vi "AlGaInPAs_prep_run_cont_v06.vi"(2 "Debug Mode":bool, 3 "Elapsed Time(s)":dbl, 4 "State":enum16{"Edit", "Start", "Run", "End", "Idle"}(ring), 5 "Argument List In":string[](array[string])) -> (0 "Status Out":string, 1 "Argument List Out":string[](array[string]))   [LabVIEW 2011]
panel:
  out "first":bool=TRUE
  out "total time":dbl
  out "is OK?":bool
  out "AsH3?":bool
  out "PH3?":bool
  out "In?":bool
  out "Ga?":bool
  out "Al?":bool
  in  "Prep As":bool caption="Pre-run"
  in  "Prep P":bool caption="Pre-run"
  in  "Prep In":bool caption="Pre-run"
  in  "Prep Ga":bool caption="Pre-run"
  in  "prep_time":dbl caption="pre-run time (s)"
  in  "Prep Al":bool caption="Pre-run"
  in  "Run As":bool caption="Run"
  in  "AsH3 Flow":dbl caption="AsH3 Flow (0-10 sccm)" format="%.2f"
  in  "P Flow":dbl caption="P Flow (0-100 sccm)" format="%.2f"
  in  "Run P":bool caption="Run"
  in  "In Flow":dbl caption="In Flow (0-100 sscm)" format="%.2f"
  in  "Run In":bool caption="Run"
  in  "Run Ga":bool caption="Run"
  in  "Ga Flow":dbl caption="Ga Flow (0-10 sscm)" format="%.2f"
  in  "Run Al":bool caption="Run"
  in  "Al Flow":dbl caption="Al Flow (0-100 sscm)" format="%.2f"
  in  "Cancel":bool
  in  "OK":bool
  out "tTotal(s) 2":dbl
  # "Add pre-run time to run time in editor."
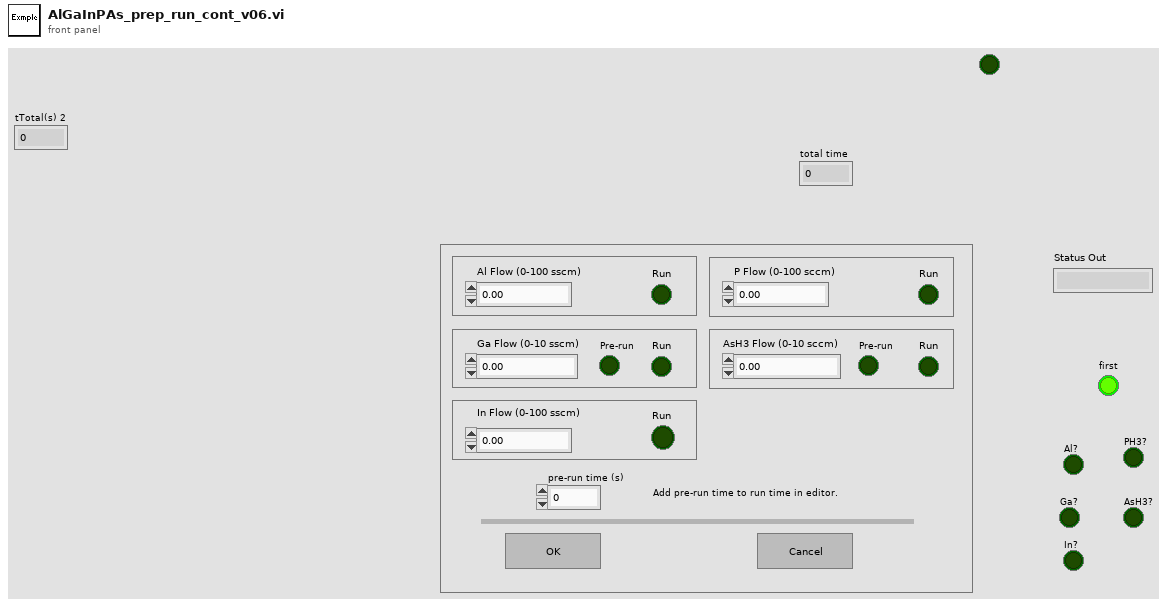
[diagram p1: front panel]
types:
  T1 = enum16{"Discrete", "Continuous", "Instantaneous"}
  T2 = enum32{"Invalid", "Default", "Floating", "Floating/Auto-Hide", "Modal"}
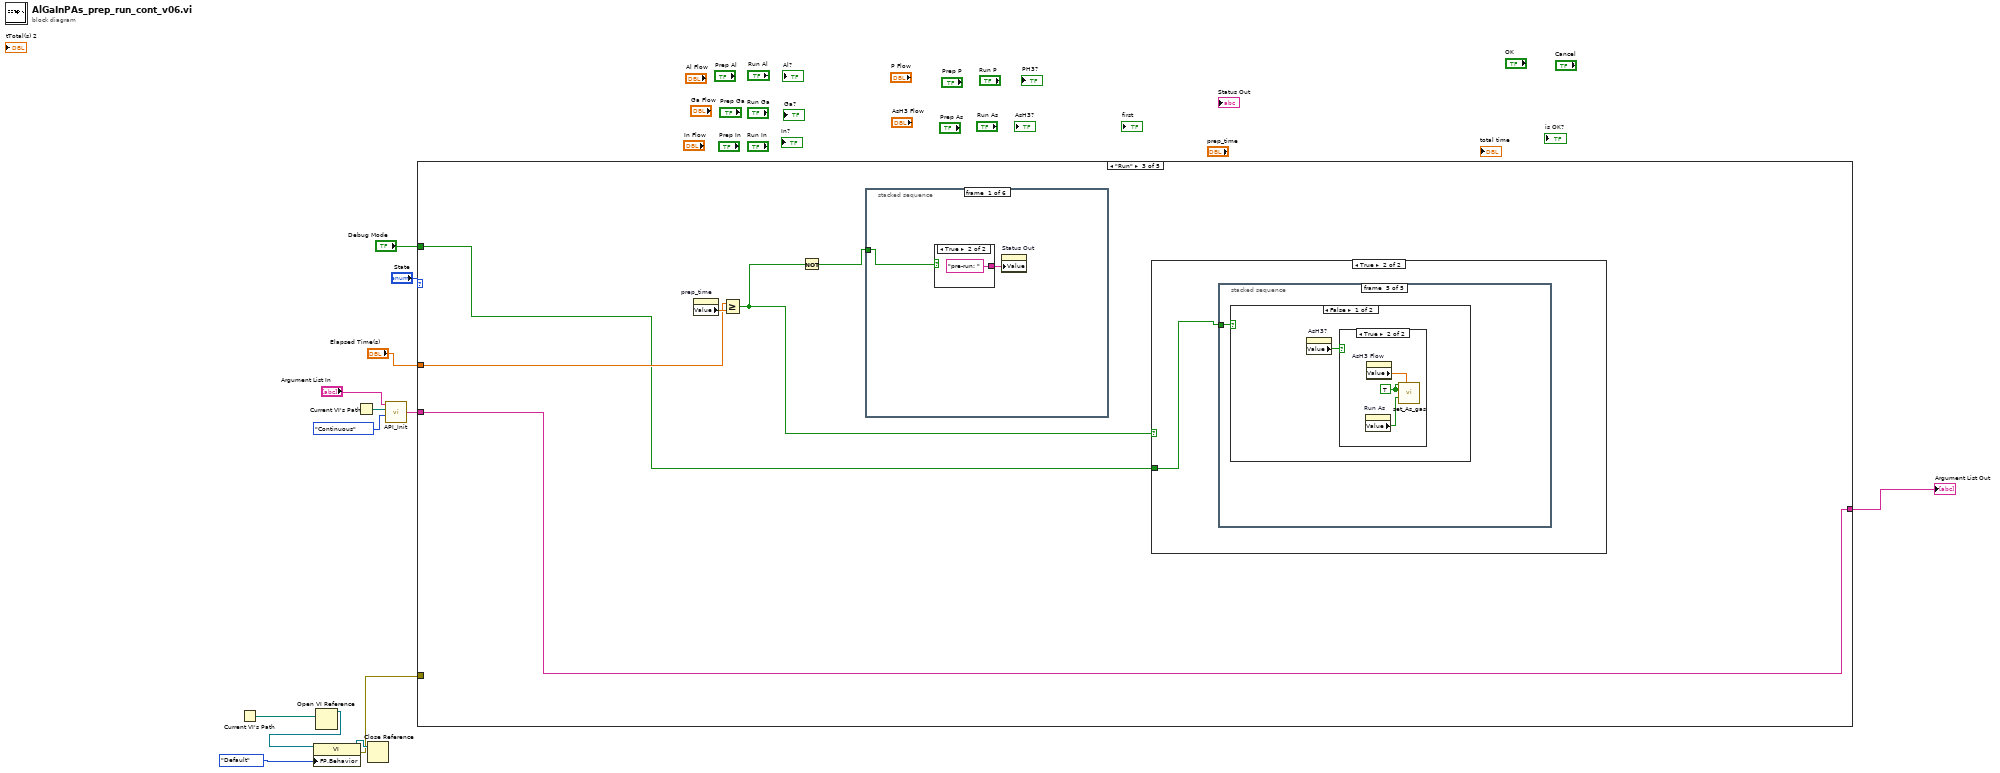
[diagram p0: block diagram]
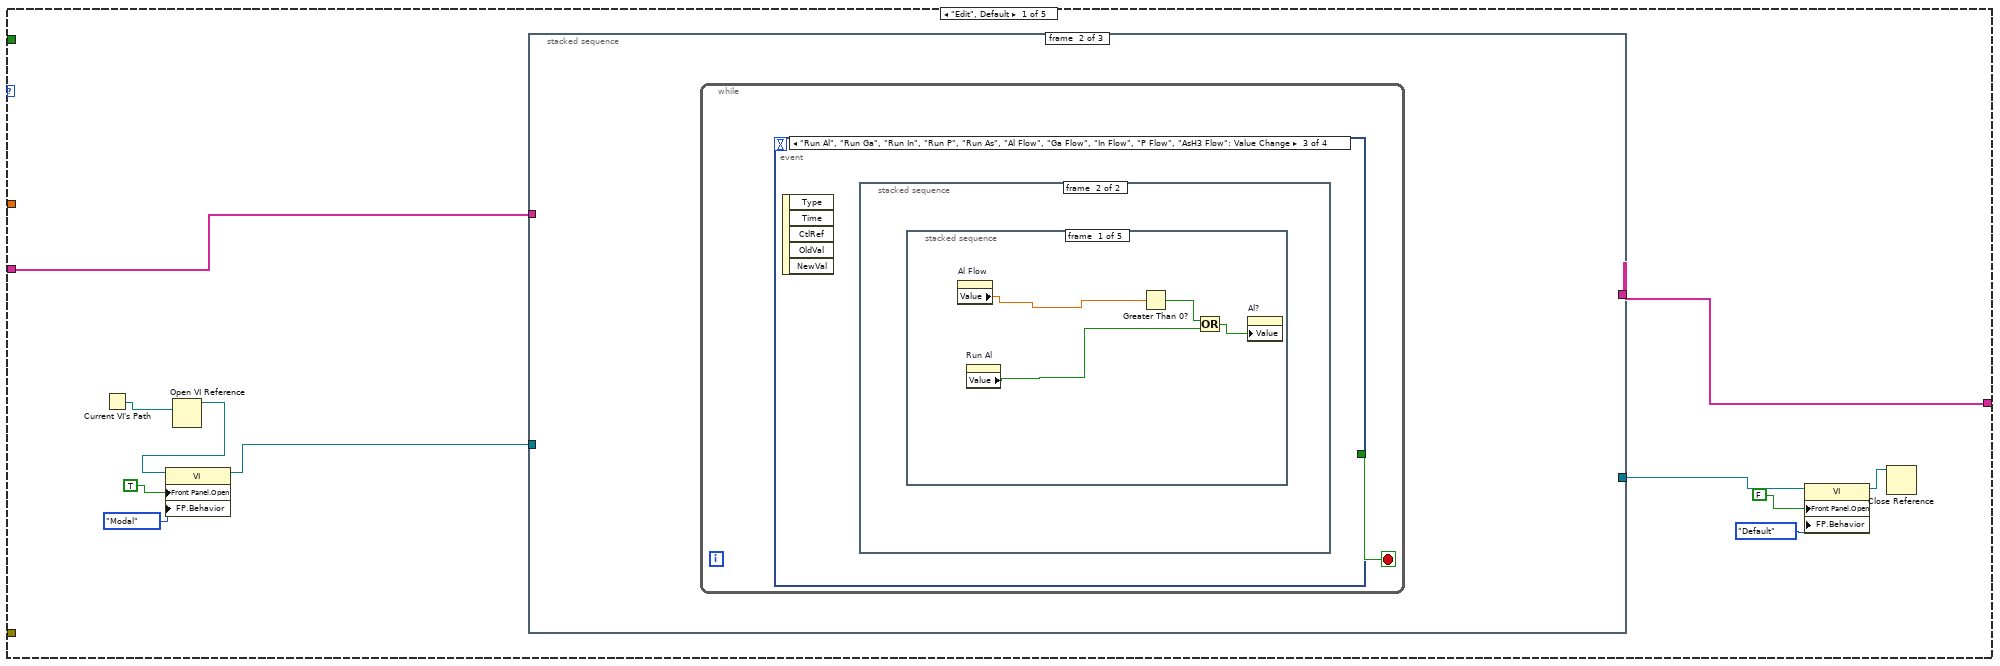
[diagram p2: hidden frame]
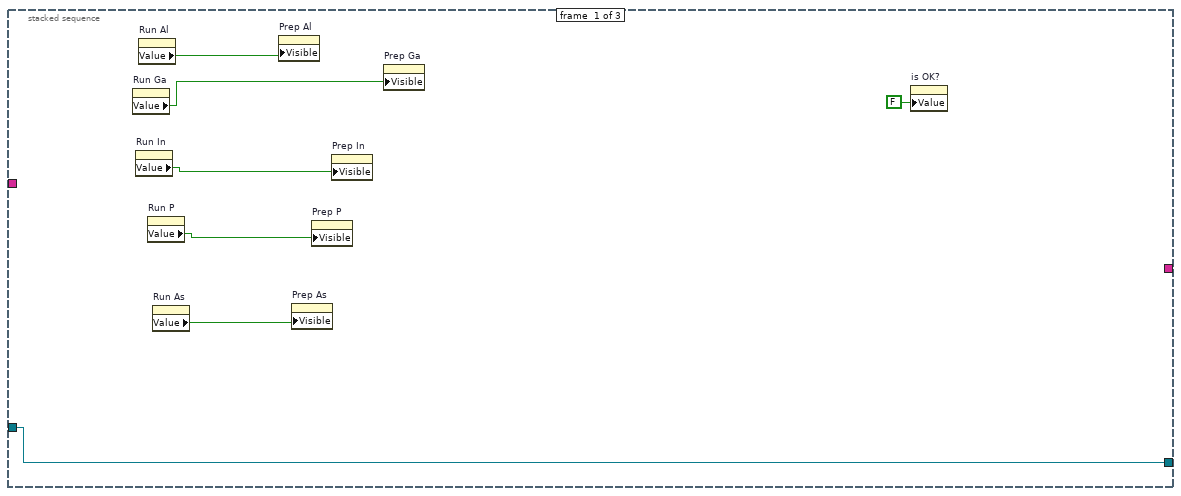
[diagram p3: hidden frame]
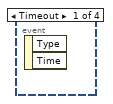
[diagram p4: hidden frame]
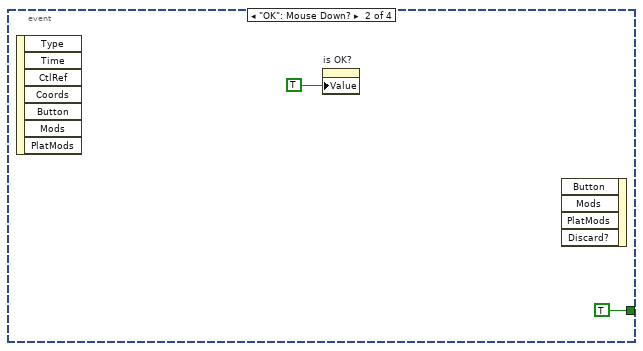
[diagram p5: hidden frame]
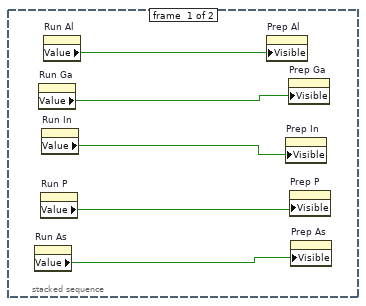
[diagram p6: hidden frame]
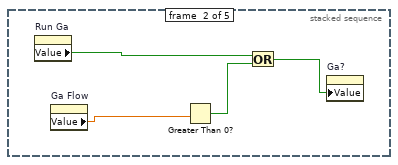
[diagram p7: hidden frame]
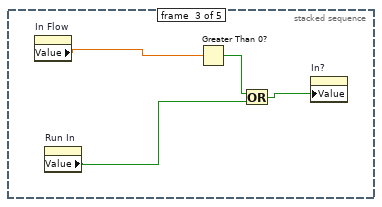
[diagram p8: hidden frame]
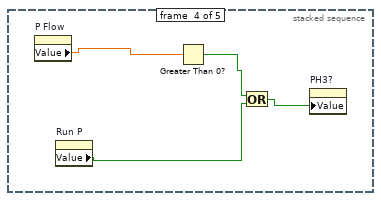
[diagram p9: hidden frame]
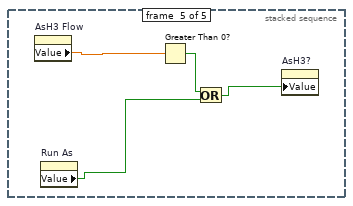
[diagram p10: hidden frame]
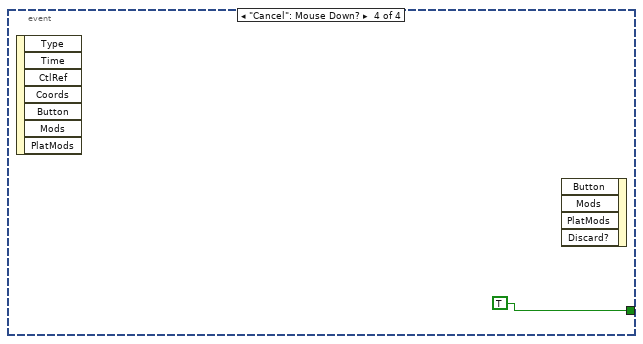
[diagram p11: hidden frame]
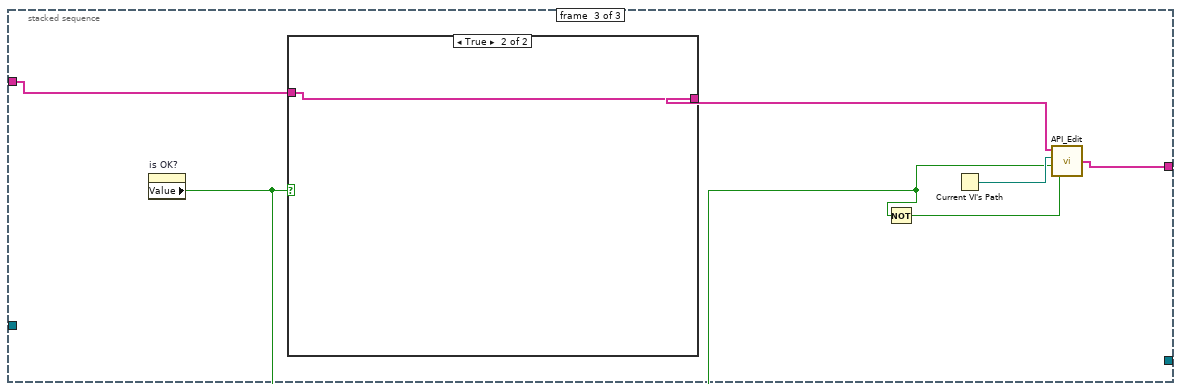
[diagram p12: hidden frame]
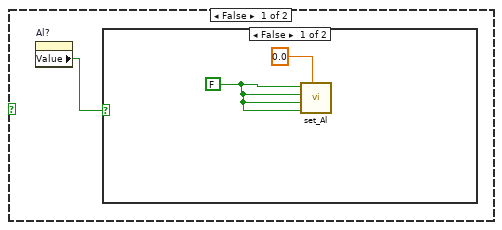
[diagram p15: hidden frame]
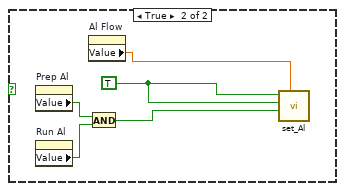
[diagram p16: hidden frame]
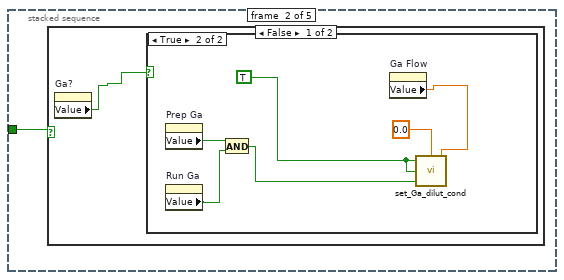
[diagram p17: hidden frame]
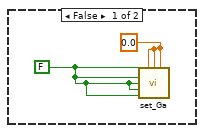
[diagram p18: hidden frame]
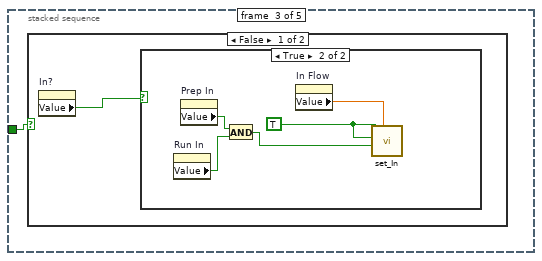
[diagram p20: hidden frame]
diagram:
  n1 = Current VI's Path() -> (path=w9:path)
  n2 = Open VI Reference(vi path=w9) -> (vi reference=w8:refnum<vi>)  [unwired: 1 in, 5 out]
  n3 = property class="VI"(reference=w8, "FP.Behavior"=T2."Default" ("Front Panel Window:Behavior")) -> (reference out=w6:refnum<vi>, error out=w5:errorcluster)  [unwired: 1 in]
  n4 = Current VI's Path() -> (path=w4:path)
  n5 = Close Reference(reference=w6) -> ()  [unwired: 1 in, 1 out]
  n6 = call "API_Init.vi"("API Mode"=T1."Continuous", "VI Path"=w4, "Argument List In"="Argument List In") -> ("Argument List Out"=w1:string[])  [unwired: 1 in]
  n7 = case shown="\"Run\"" "State" {
    tunnel: "Debug Mode" -> [_ w69 w120 _ _]
    tunnel: "Elapsed Time(s)" -> [_ _ w121 _ _]
    tunnel: w1 -> [w15 w70 w123 w210 w211]
    tunnel: [w14 w70 w123 w210 w211] -> w10
    tunnel: w5 -> [_ _ _ _ _]
    frame "Edit", Default {
      n8 = Current VI's Path() -> (path=w20:path)
      n9 = Open VI Reference(vi path=w20) -> (vi reference=w19:refnum<vi>)  [unwired: 1 in, 5 out]
      n10 = property class="VI"(reference=w19, "Front Panel.Open"=TRUE ("Front Panel Window:Open"), "FP.Behavior"=T2."Modal" ("Front Panel Window:Behavior")) -> (reference out=w18:refnum<vi>)  [unwired: 1 in, 1 out]
      n11 = stacked-sequence {
        tunnel: w15 -> [_ _ w64]
        tunnel: w18 -> [w31 _ _]
        tunnel: [w31 _ _] -> w22
        tunnel: [_ _ w62] -> w14
        frame #0 {
          n12 = property on="Run Ga" class="Bool (strict)"() -> ("Value"=w28:bool)  [unwired: 2 in, 2 out]
          n13 = property on="Run In" class="Bool (strict)"() -> ("Value"=w27:bool)  [unwired: 2 in, 2 out]
          n14 = property on="Run Al" class="Bool (strict)"() -> ("Value"=w29:bool)  [unwired: 2 in, 2 out]
          n15 = property on="Run P" class="Bool (strict)"() -> ("Value"=w26:bool)  [unwired: 2 in, 2 out]
          n16 = property on="Run As" class="Bool (strict)"() -> ("Value"=w25:bool)  [unwired: 2 in, 2 out]
          n17 = property on="Prep Al" class="Bool (strict)"("Visible"=w29) -> ()  [unwired: 2 in, 2 out]
          n18 = property on="Prep As" class="Bool (strict)"("Visible"=w25) -> ()  [unwired: 2 in, 2 out]
          n19 = property on="Prep P" class="Bool (strict)"("Visible"=w26) -> ()  [unwired: 2 in, 2 out]
          n20 = property on="Prep In" class="Bool (strict)"("Visible"=w27) -> ()  [unwired: 2 in, 2 out]
          n21 = property on="Prep Ga" class="Bool (strict)"("Visible"=w28) -> ()  [unwired: 2 in, 2 out]
          n22 = property on="is OK?" class="Bool (strict)"("Value"=FALSE ("is OK?")) -> ()  [unwired: 2 in, 2 out]
        }
        frame #1 {
          n23 = while {
            stop <- w32 stop-if-true
            n24 = event shown="[2] \"Run Al\", \"Run Ga\", \"Run In\", \"Run P\", \"Run As\", \"Al Flow\", \"Ga Flow\", \"In Flow\", \"P Flow\", \"AsH3 Flow\": Value Change" {
              selector: _ -> [_ _ _ _]
              dyn-events: _ -> [_ _ _ _]
              timeout: _ -> [_ _ _ _]
              tunnel: [_ TRUE _ TRUE] -> w32
              event Timeout {
                n25 = event-data() -> ()  [unwired: 1 in, 2 out]
              }
              event "OK": Mouse Down? {
                n26 = event-data() -> ()  [unwired: 1 in, 7 out]
                n27 = property on="is OK?" class="Bool (strict)"("Value"=TRUE ("is OK?")) -> ()  [unwired: 2 in, 2 out]
                n28 = event-data() -> ()  [unwired: 5 in, 1 out]
              }
              event "Run Al", "Run Ga", "Run In", "Run P", "Run As", "Al Flow", "Ga Flow", "In Flow", "P Flow", "AsH3 Flow": Value Change {
                n29 = event-data() -> ()  [unwired: 1 in, 5 out]
                n30 = stacked-sequence {
                  frame #0 {
                    n31 = property on="Run As" class="Bool (strict)"() -> ("Value"=w35:bool)  [unwired: 2 in, 2 out]
                    n32 = property on="Run Ga" class="Bool (strict)"() -> ("Value"=w38:bool)  [unwired: 2 in, 2 out]
                    n33 = property on="Run P" class="Bool (strict)"() -> ("Value"=w36:bool)  [unwired: 2 in, 2 out]
                    n34 = property on="Run In" class="Bool (strict)"() -> ("Value"=w37:bool)  [unwired: 2 in, 2 out]
                    n35 = property on="Run Al" class="Bool (strict)"() -> ("Value"=w39:bool)  [unwired: 2 in, 2 out]
                    n36 = property on="Prep Al" class="Bool (strict)"("Visible"=w39) -> ()  [unwired: 2 in, 2 out]
                    n37 = property on="Prep In" class="Bool (strict)"("Visible"=w37) -> ()  [unwired: 2 in, 2 out]
                    n38 = property on="Prep Ga" class="Bool (strict)"("Visible"=w38) -> ()  [unwired: 2 in, 2 out]
                    n39 = property on="Prep P" class="Bool (strict)"("Visible"=w36) -> ()  [unwired: 2 in, 2 out]
                    n40 = property on="Prep As" class="Bool (strict)"("Visible"=w35) -> ()  [unwired: 2 in, 2 out]
                  }
                  frame #1 {
                    n41 = stacked-sequence {
                      frame #0 {
                        n42 = property on="Al Flow" class="DigNum (strict)"() -> ("Value"=w42:dbl)  [unwired: 2 in, 2 out]
                        n43 = property on="Run Al" class="Bool (strict)"() -> ("Value"=w41:bool)  [unwired: 2 in, 2 out]
                        n44 = Greater Than 0?(x=w42) -> (x > 0?=w43:bool)
                        n45 = Or(x=w43, y=w41) -> (x .or. y?=w40:bool)
                        n46 = property on="Al?" class="Bool (strict)"("Value"=w40) -> ()  [unwired: 2 in, 2 out]
                      }
                      frame #1 {
                        n47 = property on="Run Ga" class="Bool (strict)"() -> ("Value"=w45:bool)  [unwired: 2 in, 2 out]
                        n48 = property on="Ga Flow" class="DigNum (strict)"() -> ("Value"=w46:dbl)  [unwired: 2 in, 2 out]
                        n49 = Greater Than 0?(x=w46) -> (x > 0?=w47:bool)
                        n50 = Or(x=w45, y=w47) -> (x .or. y?=w44:bool)
                        n51 = property on="Ga?" class="Bool (strict)"("Value"=w44) -> ()  [unwired: 2 in, 2 out]
                      }
                      frame #2 {
                        n52 = property on="In Flow" class="DigNum (strict)"() -> ("Value"=w49:dbl)  [unwired: 2 in, 2 out]
                        n53 = property on="Run In" class="Bool (strict)"() -> ("Value"=w50:bool)  [unwired: 2 in, 2 out]
                        n54 = Greater Than 0?(x=w49) -> (x > 0?=w51:bool)
                        n55 = Or(x=w51, y=w50) -> (x .or. y?=w48:bool)
                        n56 = property on="In?" class="Bool (strict)"("Value"=w48) -> ()  [unwired: 2 in, 2 out]
                      }
                      frame #3 {
                        n57 = property on="P Flow" class="DigNum (strict)"() -> ("Value"=w54:dbl)  [unwired: 2 in, 2 out]
                        n58 = property on="Run P" class="Bool (strict)"() -> ("Value"=w53:bool)  [unwired: 2 in, 2 out]
                        n59 = Greater Than 0?(x=w54) -> (x > 0?=w55:bool)
                        n60 = Or(x=w55, y=w53) -> (x .or. y?=w52:bool)
                        n61 = property on="PH3?" class="Bool (strict)"("Value"=w52) -> ()  [unwired: 2 in, 2 out]
                      }
                      frame #4 {
                        n62 = property on="AsH3 Flow" class="DigNum (strict)"() -> ("Value"=w58:dbl)  [unwired: 2 in, 2 out]
                        n63 = property on="Run As" class="Bool (strict)"() -> ("Value"=w57:bool)  [unwired: 2 in, 2 out]
                        n64 = Greater Than 0?(x=w58) -> (x > 0?=w59:bool)
                        n65 = Or(x=w59, y=w57) -> (x .or. y?=w56:bool)
                        n66 = property on="AsH3?" class="Bool (strict)"("Value"=w56) -> ()  [unwired: 2 in, 2 out]
                      }
                    }
                  }
                }
              }
              event "Cancel": Mouse Down? {
                n67 = event-data() -> ()  [unwired: 1 in, 7 out]
                n68 = event-data() -> ()  [unwired: 5 in, 1 out]
              }
            }
          }
        }
        frame #2 {
          n69 = property on="is OK?" class="Bool (strict)"() -> ("Value"=w61:bool)  [unwired: 2 in, 2 out]
          n70 = case shown="True" w61 {
            tunnel: w64 -> [w67 w68]
            tunnel: [w67 w68] -> w63
            frame False {
            }
            frame True {
            }
          }
          n71 = Not(x=w61) -> (.not. x?=w66:bool)
          n72 = Current VI's Path() -> (path=w65:path)
          n73 = call "API_Edit.vi"("Cancel"=w66, "OK"=w61, "VI Path"=w65, "Argument List In"=w63) -> ("Argument List Out"=w62:string[])
        }
      }
      n74 = property class="VI"(reference=w22, "Front Panel.Open"=FALSE ("Front Panel Window:Open"), "FP.Behavior"=T2."Default" ("Front Panel Window:Behavior")) -> (reference out=w23:refnum<vi>)  [unwired: 1 in, 1 out]
      n75 = Close Reference(reference=w23) -> ()  [unwired: 1 in, 1 out]
    }
    frame "Start" {
      n76 = stacked-sequence {
        tunnel: w69 -> [w71]
        frame #0 {
          n77 = stacked-sequence {
            tunnel: w71 -> [w72 w81 w91 w100 w109]
            frame #0 {
              n78 = case shown="True" w72 {
                frame False {
                  n79 = property on="Al?" class="Bool (strict)"() -> ("Value"=w73:bool)  [unwired: 2 in, 2 out]
                  n80 = case shown="False" w73 {
                    frame False {
                      w74 = FALSE ("Al Active")
                      n81 = call "set_Al.vi"("Aluminum Flow"=0.0, "Al Remote"=w74, "Al Run"=w74, "Al Bubbler"=w74, "Al Active"=w74) -> ()  [unwired: 5 out]
                    }
                    frame True {
                      w80 = TRUE ("Al Active")
                      n82 = property on="Prep Al" class="Bool (strict)"() -> ("Value"=w78:bool)  [unwired: 2 in, 2 out]
                      n83 = property on="Run Al" class="Bool (strict)"() -> ("Value"=w77:bool)  [unwired: 2 in, 2 out]
                      n84 = property on="Al Flow" class="DigNum (strict)"() -> ("Value"=w79:dbl)  [unwired: 2 in, 2 out]
                      n85 = And(x=w78, y=w77) -> (x .and. y?=w76:bool)
                      n86 = call "set_Al.vi"("Aluminum Flow"=w79, "Al Run"=w76, "Al Bubbler"=w80, "Al Active"=w80) -> ()  [unwired: 1 in, 5 out]
                    }
                  }
                }
                frame True {
                }
              }
            }
            frame #1 {
              n87 = case shown="False" w81 {
                frame False {
                  n88 = property on="Ga?" class="Bool (strict)"() -> ("Value"=w82:bool)  [unwired: 2 in, 2 out]
                  n89 = case shown="True" w82 {
                    frame False {
                      w84 = FALSE ("Ga Active")
                      w83 = 0.0 ("Ga Flow 1")
                      n90 = call "set_Ga.vi"("Ga Active"=w84, "Ga Flow 3"=w83, "Ga Flow 2"=w83, "Ga Flow 1"=w83, "Ga Bubbler"=w84, "Ga H2 Dilute"=w84, "Ga Run"=w84, "Ga Remote"=w84) -> ()  [unwired: 8 out]
                    }
                    frame True {
                      w90 = TRUE ("Ga Active")
                      n91 = property on="Prep Ga" class="Bool (strict)"() -> ("Value"=w87:bool)  [unwired: 2 in, 2 out]
                      n92 = property on="Run Ga" class="Bool (strict)"() -> ("Value"=w86:bool)  [unwired: 2 in, 2 out]
                      n93 = And(x=w87, y=w86) -> (x .and. y?=w85:bool)
                      n94 = property on="Ga Flow" class="DigNum (strict)"() -> ("Value"=w88:dbl)  [unwired: 2 in, 2 out]
                      n95 = call "set_Ga_dilut_cond.vi"("Ga flow (0-10 sccm)"=w88, "fDilution"=0.0, "Run"=w85, "Bubbler In"=w90, "Active"=w90) -> ()
                    }
                  }
                }
                frame True {
                }
              }
            }
            frame #2 {
              n96 = case shown="False" w91 {
                frame False {
                  n97 = property on="In?" class="Bool (strict)"() -> ("Value"=w92:bool)  [unwired: 2 in, 2 out]
                  n98 = case shown="True" w92 {
                    frame False {
                      w94 = FALSE ("In Remote")
                      n99 = call "set_In.vi"("Indium Flow"=0.0, "In Remote"=w94, "In Run"=w94, "In Bubbler"=w94, "In Active"=w94) -> ()  [unwired: 5 out]
                    }
                    frame True {
                      w99 = TRUE ("In Run")
                      n100 = property on="Run In" class="Bool (strict)"() -> ("Value"=w96:bool)  [unwired: 2 in, 2 out]
                      n101 = property on="Prep In" class="Bool (strict)"() -> ("Value"=w97:bool)  [unwired: 2 in, 2 out]
                      n102 = And(x=w97, y=w96) -> (x .and. y?=w95:bool)
                      n103 = property on="In Flow" class="DigNum (strict)"() -> ("Value"=w98:dbl)  [unwired: 2 in, 2 out]
                      n104 = call "set_In.vi"("Indium Flow"=w98, "In Run"=w95, "In Bubbler"=w99, "In Active"=w99) -> ()  [unwired: 1 in, 5 out]
                    }
                  }
                }
                frame True {
                }
              }
            }
            frame #3 {
              n105 = case shown="False" w100 {
                frame False {
                  n106 = property on="PH3?" class="Bool (strict)"() -> ("Value"=w101:bool)  [unwired: 2 in, 2 out]
                  n107 = case shown="True" w101 {
                    frame False {
                      w102 = FALSE ("P_Gas Active")
                      n108 = call "set_P_gas.vi"("P_Gas Active"=w102, "P_Gas Flow"=0.0, "P_Gas In"=w102, "P_Gas H2 In"=w102, "P_Gas Run"=w102, "P_Gas Remote"=w102) -> ()  [unwired: 10 out]
                    }
                    frame True {
                      w108 = TRUE ("P_Gas Active")
                      n109 = property on="P Flow" class="DigNum (strict)"() -> ("Value"=w107:dbl)  [unwired: 2 in, 2 out]
                      n110 = property on="Prep P" class="Bool (strict)"() -> ("Value"=w106:bool)  [unwired: 2 in, 2 out]
                      n111 = property on="Run P" class="Bool (strict)"() -> ("Value"=w105:bool)  [unwired: 2 in, 2 out]
                      n112 = And(x=w106, y=w105) -> (x .and. y?=w104:bool)
                      n113 = call "set_P_gas.vi"("P_Gas Active"=w108, "P_Gas Flow"=w107, "P_Gas In"=w108, "P_Gas Run"=w104) -> ()  [unwired: 2 in, 10 out]
                    }
                  }
                }
                frame True {
                }
              }
            }
            frame #4 {
              n114 = case shown="False" w109 {
                frame False {
                  n115 = property on="AsH3?" class="Bool (strict)"() -> ("Value"=w110:bool)  [unwired: 2 in, 2 out]
                  n116 = case shown="True" w110 {
                    frame False {
                      w111 = FALSE ("As_Gas Active")
                      n117 = call "set_As_gas.vi"("As_Gas Active"=w111, "As_Gas Flow"=0.0, "As_Gas In"=w111, "As_Gas H2"=w111, "As_Gas Run"=w111, "As_Gas Remote"=w111) -> ()  [unwired: 10 in]
                    }
                    frame True {
                      w117 = TRUE ("As_Gas Active")
                      n118 = property on="Prep As" class="Bool (strict)"() -> ("Value"=w114:bool)  [unwired: 2 in, 2 out]
                      n119 = property on="Run As" class="Bool (strict)"() -> ("Value"=w115:bool)  [unwired: 2 in, 2 out]
                      n120 = property on="AsH3 Flow" class="DigNum (strict)"() -> ("Value"=w116:dbl)  [unwired: 2 in, 2 out]
                      n121 = And(x=w114, y=w115) -> (x .and. y?=w113:bool)
                      n122 = call "set_As_gas.vi"("As_Gas Active"=w117, "As_Gas Flow"=w116, "As_Gas In"=w117, "As_Gas Run"=w113) -> ()  [unwired: 12 in]
                    }
                  }
                }
                frame True {
                }
              }
            }
          }
        }
      }
    }
    frame "Run" {
      n123 = property on="prep_time" class="DigNum (strict)"() -> ("Value"=w122:dbl)  [unwired: 2 in, 2 out]
      n124 = Greater Or Equal?(x=w121, y=w122) -> (x >= y?=w119:bool)
      n125 = Not(x=w119) -> (.not. x?=w118:bool)
      n126 = stacked-sequence {
        tunnel: w118 -> [w125 w129 w138 w147 w156 w165]
        frame #0 {
          n127 = case shown="True" w125 {
            tunnel: ["run: " "pre-run: "] -> w124
            frame False {
            }
            frame True {
            }
          }
          n128 = property on="Status Out" class="Str"("Value"=w124) -> ()  [unwired: 2 in, 2 out]
        }
        frame #1 {
          n129 = property on="Status Out" class="Str"() -> ("Value"=w135:string)  [unwired: 2 in, 2 out]
          n130 = property on="Al?" class="Bool (strict)"() -> ("Value"=w136:bool)  [unwired: 2 in, 2 out]
          n131 = property on="Run Al" class="Bool (strict)"() -> ("Value"=w128:bool)  [unwired: 2 in, 2 out]
          n132 = property on="Prep Al" class="Bool (strict)"() -> ("Value"=w130:bool)  [unwired: 2 in, 2 out]
          n133 = call "flow_strings.vi"("string in"=w135, "is first in?"=TRUE, "use source?"=w136, "name"="Al", "run source?"=w128, "prep source?"=w130, "is prep?"=w129) -> ("string out"=w134:string, "is first out?"=w133:bool)
          n134 = property on="Status Out" class="Str"("Value"=w134) -> ()  [unwired: 2 in, 2 out]
          n135 = property on="first" class="Bool (strict)"("Value"=w133) -> ()  [unwired: 2 in, 2 out]
        }
        frame #2 {
          n136 = property on="first" class="Bool (strict)"() -> ("Value"=w141:bool)  [unwired: 2 in, 2 out]
          n137 = property on="Status Out" class="Str"() -> ("Value"=w144:string)  [unwired: 2 in, 2 out]
          n138 = property on="Ga?" class="Bool (strict)"() -> ("Value"=w142:bool)  [unwired: 2 in, 2 out]
          n139 = property on="Run Ga" class="Bool (strict)"() -> ("Value"=w137:bool)  [unwired: 2 in, 2 out]
          n140 = property on="Prep Ga" class="Bool (strict)"() -> ("Value"=w139:bool)  [unwired: 2 in, 2 out]
          n141 = call "flow_strings.vi"("string in"=w144, "is first in?"=w141, "use source?"=w142, "name"="Ga", "run source?"=w137, "prep source?"=w139, "is prep?"=w138) -> ("string out"=w145:string, "is first out?"=w140:bool)
          n142 = property on="Status Out" class="Str"("Value"=w145) -> ()  [unwired: 2 in, 2 out]
          n143 = property on="first" class="Bool (strict)"("Value"=w140) -> ()  [unwired: 2 in, 2 out]
        }
        frame #3 {
          n144 = property on="first" class="Bool (strict)"() -> ("Value"=w151:bool)  [unwired: 2 in, 2 out]
          n145 = property on="Status Out" class="Str"() -> ("Value"=w153:string)  [unwired: 2 in, 2 out]
          n146 = property on="In?" class="Bool (strict)"() -> ("Value"=w154:bool)  [unwired: 2 in, 2 out]
          n147 = property on="Run In" class="Bool (strict)"() -> ("Value"=w146:bool)  [unwired: 2 in, 2 out]
          n148 = property on="Prep In" class="Bool (strict)"() -> ("Value"=w148:bool)  [unwired: 2 in, 2 out]
          n149 = call "flow_strings.vi"("string in"=w153, "is first in?"=w151, "use source?"=w154, "name"="In", "run source?"=w146, "prep source?"=w148, "is prep?"=w147) -> ("string out"=w150:string, "is first out?"=w149:bool)
          n150 = property on="Status Out" class="Str"("Value"=w150) -> ()  [unwired: 2 in, 2 out]
          n151 = property on="first" class="Bool (strict)"("Value"=w149) -> ()  [unwired: 2 in, 2 out]
        }
        frame #4 {
          n152 = property on="first" class="Bool (strict)"() -> ("Value"=w159:bool)  [unwired: 2 in, 2 out]
          n153 = property on="Status Out" class="Str"() -> ("Value"=w161:string)  [unwired: 2 in, 2 out]
          n154 = property on="PH3?" class="Bool (strict)"() -> ("Value"=w162:bool)  [unwired: 2 in, 2 out]
          n155 = property on="Run P" class="Bool (strict)"() -> ("Value"=w155:bool)  [unwired: 2 in, 2 out]
          n156 = property on="Prep P" class="Bool (strict)"() -> ("Value"=w157:bool)  [unwired: 2 in, 2 out]
          n157 = call "flow_strings.vi"("string in"=w161, "is first in?"=w159, "use source?"=w162, "name"="P", "run source?"=w155, "prep source?"=w157, "is prep?"=w156) -> ("string out"=w160:string, "is first out?"=w158:bool)
          n158 = property on="Status Out" class="Str"("Value"=w160) -> ()  [unwired: 2 in, 2 out]
          n159 = property on="first" class="Bool (strict)"("Value"=w158) -> ()  [unwired: 2 in, 2 out]
        }
        frame #5 {
          n160 = property on="first" class="Bool (strict)"() -> ("Value"=w168:bool)  [unwired: 2 in, 2 out]
          n161 = property on="Status Out" class="Str"() -> ("Value"=w170:string)  [unwired: 2 in, 2 out]
          n162 = property on="AsH3?" class="Bool (strict)"() -> ("Value"=w171:bool)  [unwired: 2 in, 2 out]
          n163 = property on="Run As" class="Bool (strict)"() -> ("Value"=w164:bool)  [unwired: 2 in, 2 out]
          n164 = property on="Prep As" class="Bool (strict)"() -> ("Value"=w166:bool)  [unwired: 2 in, 2 out]
          n165 = call "flow_strings.vi"("string in"=w170, "is first in?"=w168, "use source?"=w171, "name"="As", "run source?"=w164, "prep source?"=w166, "is prep?"=w165) -> ("string out"=w167:string, "is first out?"=w169:bool)
          n166 = property on="Status Out" class="Str"("Value"=w167) -> ()  [unwired: 2 in, 2 out]
          n167 = property on="first" class="Bool (strict)"("Value"=w169) -> ()  [unwired: 2 in, 2 out]
        }
      }
      n168 = case shown="True" w119 {
        tunnel: w120 -> [_ w173]
        frame False {
        }
        frame True {
          n169 = stacked-sequence {
            tunnel: w173 -> [w174 w181 w189 w196 w203]
            frame #0 {
              n170 = case shown="True" w174 {
                frame False {
                  n171 = property on="Al?" class="Bool (strict)"() -> ("Value"=w175:bool)  [unwired: 2 in, 2 out]
                  n172 = case shown="True" w175 {
                    frame False {
                      w176 = FALSE ("Al Active")
                      n173 = call "set_Al.vi"("Aluminum Flow"=0.0, "Al Remote"=w176, "Al Run"=w176, "Al Bubbler"=w176, "Al Active"=w176) -> ()  [unwired: 5 out]
                    }
                    frame True {
                      w180 = TRUE ("Al Active")
                      n174 = property on="Al Flow" class="DigNum (strict)"() -> ("Value"=w179:dbl)  [unwired: 2 in, 2 out]
                      n175 = property on="Run Al" class="Bool (strict)"() -> ("Value"=w178:bool)  [unwired: 2 in, 2 out]
                      n176 = call "set_Al.vi"("Aluminum Flow"=w179, "Al Run"=w178, "Al Bubbler"=w180, "Al Active"=w180) -> ()  [unwired: 1 in, 5 out]
                    }
                  }
                }
                frame True {
                }
              }
            }
            frame #1 {
              n177 = case shown="False" w181 {
                frame False {
                  n178 = property on="Ga?" class="Bool (strict)"() -> ("Value"=w182:bool)  [unwired: 2 in, 2 out]
                  n179 = case shown="False" w182 {
                    frame False {
                      w184 = FALSE ("Ga Active")
                      w183 = 0.0 ("Ga Flow 1")
                      n180 = call "set_Ga.vi"("Ga Active"=w184, "Ga Flow 3"=w183, "Ga Flow 2"=w183, "Ga Flow 1"=w183, "Ga Bubbler"=w184, "Ga H2 Dilute"=w184, "Ga Run"=w184, "Ga Remote"=w184) -> ()  [unwired: 8 out]
                    }
                    frame True {
                      w188 = TRUE ("Ga Active")
                      n181 = property on="Ga Flow" class="DigNum (strict)"() -> ("Value"=w185:dbl)  [unwired: 2 in, 2 out]
                      n182 = property on="Run Ga" class="Bool (strict)"() -> ("Value"=w186:bool)  [unwired: 2 in, 2 out]
                      n183 = call "set_Ga_dilut_cond.vi"("Ga flow (0-10 sccm)"=w185, "fDilution"=0.0, "Run"=w186, "Bubbler In"=w188, "Active"=w188) -> ()
                    }
                  }
                }
                frame True {
                }
              }
            }
            frame #2 {
              n184 = case shown="False" w189 {
                frame False {
                  n185 = property on="In?" class="Bool (strict)"() -> ("Value"=w190:bool)  [unwired: 2 in, 2 out]
                  n186 = case shown="True" w190 {
                    frame False {
                      w192 = FALSE ("In Remote")
                      n187 = call "set_In.vi"("Indium Flow"=0.0, "In Remote"=w192, "In Run"=w192, "In Bubbler"=w192, "In Active"=w192) -> ()  [unwired: 5 out]
                    }
                    frame True {
                      w195 = TRUE ("In Run")
                      n188 = property on="Run In" class="Bool (strict)"() -> ("Value"=w193:bool)  [unwired: 2 in, 2 out]
                      n189 = property on="In Flow" class="DigNum (strict)"() -> ("Value"=w194:dbl)  [unwired: 2 in, 2 out]
                      n190 = call "set_In.vi"("Indium Flow"=w194, "In Run"=w193, "In Bubbler"=w195, "In Active"=w195) -> ()  [unwired: 1 in, 5 out]
                    }
                  }
                }
                frame True {
                }
              }
            }
            frame #3 {
              n191 = case shown="False" w196 {
                frame False {
                  n192 = property on="PH3?" class="Bool (strict)"() -> ("Value"=w197:bool)  [unwired: 2 in, 2 out]
                  n193 = case shown="False" w197 {
                    frame False {
                      w198 = FALSE ("P_Gas Active")
                      n194 = call "set_P_gas.vi"("P_Gas Active"=w198, "P_Gas Flow"=0.0, "P_Gas In"=w198, "P_Gas H2 In"=w198, "P_Gas Run"=w198, "P_Gas Remote"=w198) -> ()  [unwired: 10 out]
                    }
                    frame True {
                      w202 = TRUE ("P_Gas Active")
                      n195 = property on="P Flow" class="DigNum (strict)"() -> ("Value"=w201:dbl)  [unwired: 2 in, 2 out]
                      n196 = property on="Run P" class="Bool (strict)"() -> ("Value"=w200:bool)  [unwired: 2 in, 2 out]
                      n197 = call "set_P_gas.vi"("P_Gas Active"=w202, "P_Gas Flow"=w201, "P_Gas In"=w202, "P_Gas Run"=w200) -> ()  [unwired: 2 in, 10 out]
                    }
                  }
                }
                frame True {
                }
              }
            }
            frame #4 {
              n198 = case shown="False" w203 {
                frame False {
                  n199 = property on="AsH3?" class="Bool (strict)"() -> ("Value"=w204:bool)  [unwired: 2 in, 2 out]
                  n200 = case shown="True" w204 {
                    frame False {
                      w205 = FALSE ("As_Gas Active")
                      n201 = call "set_As_gas.vi"("As_Gas Active"=w205, "As_Gas Flow"=0.0, "As_Gas In"=w205, "As_Gas H2"=w205, "As_Gas Run"=w205, "As_Gas Remote"=w205) -> ()  [unwired: 10 in]
                    }
                    frame True {
                      w208 = TRUE ("As_Gas Active")
                      n202 = property on="Run As" class="Bool (strict)"() -> ("Value"=w207:bool)  [unwired: 2 in, 2 out]
                      n203 = property on="AsH3 Flow" class="DigNum (strict)"() -> ("Value"=w209:dbl)  [unwired: 2 in, 2 out]
                      n204 = call "set_As_gas.vi"("As_Gas Active"=w208, "As_Gas Flow"=w209, "As_Gas In"=w208, "As_Gas Run"=w207) -> ()  [unwired: 12 in]
                    }
                  }
                }
                frame True {
                }
              }
            }
          }
        }
      }
    }
    frame "End" {
    }
    frame "Idle" {
    }
  }
  "Argument List Out" <- w10
